vi "dfd_Group Delay_Generate Design Info.vi"(4 "radius":dbl=1.0, 5 "Add Band?":bool, 6 "fs [Hz]":dbl=1.0 format="%.2f", 7 "grid density":i32=20, 8 "error in (no error)":errorcluster, 9 "p":i32=2, 10 "band specification":T2[](array[typedef]) {"subband specs"."weight" format="%.2f"}, 11 "order":i32) -> (0 "error out":errorcluster, 3 "Group Delay Design Info":T1={"p"=2, "freq grid"=[], "d"=[], "weight"=[], "Order"=0, "radius"=0.0})   [LabVIEW 2017, in "NI_DigFilter_Design.lvlib"]
uses:
  <vilib>/addons/Digital Filter Design/NI_DigFilter_Design.lvlib
  <vilib>/addons/Digital Filter Design/_GroupDelay.llb/dfd_Group Delay_Band Spec.ctl
  <vilib>/addons/Digital Filter Design/_GroupDelay.llb/dfd_Group Delay_Design Info.ctl
  <vilib>/addons/Digital Filter Design/NI_DigFilterLicensed.lvlib
panel:
  in  "Group Delay Design Info 2":T1={"p"=2, "freq grid"=[], "d"=[], "weight"=[], "Order"=0, "radius"=0.0}
  # "freq"
  # "group delay"
  # "weight"
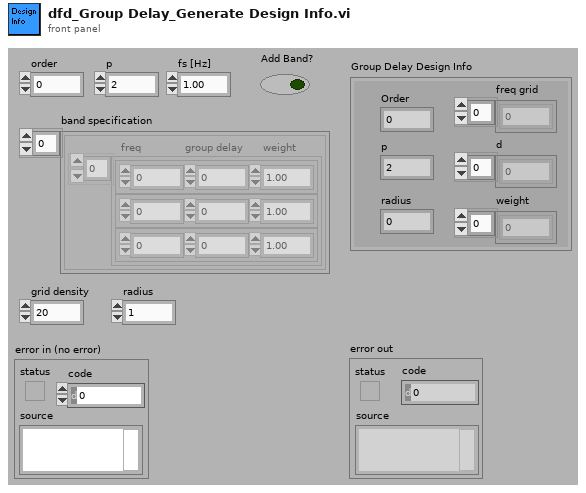
[diagram p1: front panel]
types:
  T1 = typedef "dfd_Group Delay_Design Info.ctl" = cluster{"p":i32, "freq grid":dbl[], "d":dbl[], "weight":dbl[], "Order":i32, "radius":dbl}
  T2 = typedef "NI_DigFilterLicensed.lvlib/dfd_Group Delay_Band Spec.ctl" = cluster{"subband specs":cluster{"freq":dbl, "group delay":dbl, "weight":dbl}[]}
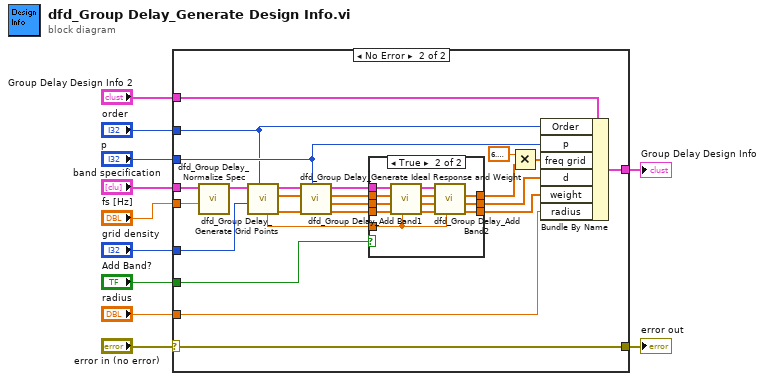
[diagram p0: block diagram]
diagram:
  n1 = case shown="No Error" "error in (no error)" {
    selector: "error in (no error)" -> [w12 w24]
    tunnel: "band specification" -> [_ w36]
    tunnel: "fs [Hz]" -> [_ w35]
    tunnel: "order" -> [_ w16]
    tunnel: "p" -> [_ w33]
    tunnel: "Add Band?" -> [_ w31]
    tunnel: "Group Delay Design Info 2" -> [_ w27]
    tunnel: [_ w26] -> w5
    tunnel: "radius" -> [_ w25]
    tunnel: [w12 w24] -> w2
    tunnel: "grid density" -> [_ w14]
    frame Error {
    }
    frame No Error {
      n2 = call <vilib>:"dfd_Group Delay_Normalize Spec.vi"("fs [Hz]"=w35, "Band"=w36) -> ("Normalized Band"=w15:T2[])  [unwired: 9 out]
      n3 = call <vilib>:"dfd_Group Delay_Generate Grid Points.vi"("Order"=w16, "grid density"=w14, "band specification"=w15) -> ("weight for grid"=w19:dbl[], "fgrid"=w18:dbl[], "band specification (dup)"=w17:T2[], "grid length"=w13:dbl)  [unwired: 5 out]
      n4 = call <vilib>:"dfd_Group Delay_Generate Ideal Response and Weight.vi"("p"=w33, "weight for grid"=w19, "fgrid"=w18, "band specification"=w17) -> ("weight"=w23:dbl[], "desired response"=w22:dbl[], "fgrid (dup)"=w21:dbl[], "band specification (dup)"=w20:T2[])  [unwired: 1 in, 3 out]
      n5 = case shown="True" w31 {
        tunnel: w21 -> [w39 w50]
        tunnel: [w39 w46] -> w30
        tunnel: [w37 w45] -> w29
        tunnel: [w38 w44] -> w28
        tunnel: w23 -> [w38 w43]
        tunnel: w22 -> [w37 w42]
        tunnel: w20 -> [_ w41]
        tunnel: w13 -> [_ w40]
        frame False {
        }
        frame True {
          n6 = call <vilib>:"dfd_Group Delay_Add Band1.vi"("grid length"=w40, "weight (in)"=w43, "d (in)"=w42, "freq grid (in)"=w50, "allpass band spec"=w41) -> ("weight (out)"=w47:dbl[], "d (out)"=w48:dbl[], "freq grid (out)"=w49:dbl[], "allpass band spec (dup)"=w51:T2[])  [unwired: 3 out]
          n7 = call <vilib>:"dfd_Group Delay_Add Band2.vi"("grid length"=w40, "weight (in)"=w47, "d (in)"=w48, "freq grid (in)"=w49, "Allpass_Band Spec"=w51) -> ("weight  (out)"=w44:dbl[], "d  (out)"=w45:dbl[], "freq grid (out)"=w46:dbl[])  [unwired: 4 out]
        }
      }
      n8 = Multiply(x=6.283185307179586, y=w30) -> (x*y=w32:dbl[])
      n9 = Bundle By Name(cluster=w27, "Order"=w16, "p"=w33, "freq grid"=w32, "d"=w29, "weight"=w28, "radius"=w25) -> (w26:T1)
    }
  }
  "error out" <- w2
  "Group Delay Design Info" <- w5
